vi "Repeat_Meas_if_Unsteady.vi"() -> (5 "Plug in titles":string[](array[string]), 7 "Plug in values":string[](array[string]))   [LabVIEW 2014]
uses:
  Controls/Post_Process.ctl
  Globals/Meas_global.vi
  <vilib>/Analysis/NI_AALPro.lvlib
panel:
  out "Waveform Graph":cluster{dbl, dbl, "Downsampled Array":dbl[][]}(graph)
  out "Repeat Measurement":bool
  in  "Minumum value to divide by":dbl=100.0 format="%#_13g"
  in  "Acceptable % Drift":dbl=0.8 format="%#_13g"
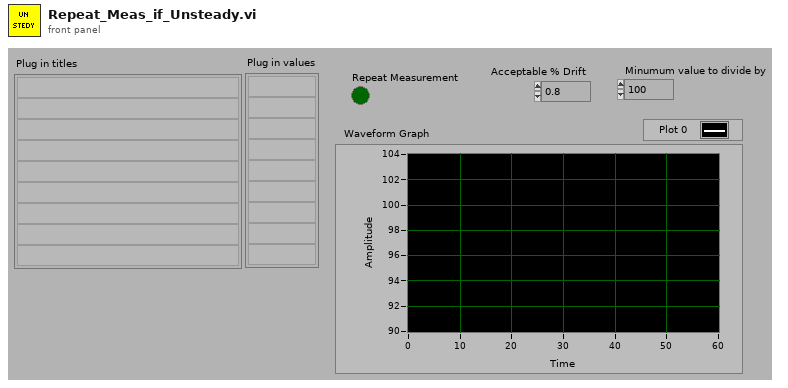
[diagram p1: front panel]
types:
  T1 = typedef "Analysis_info_cluster.ctl" = cluster{"Colour":u32, "Inst type":T2, "Inst name":string, "Symbol":string, "Code name":string, "Extra Info":string, "Inst Array":T3, "Extra Titles":string[], "Extra Values":string[], "U":dbl, "u^2":dbl, "u^3":dbl, "u^4":dbl, "Skew_u":dbl, "Kurt_u":dbl, "Sd Error in Mean":dbl, "% u'/U":dbl, "X":dbl, "Y":dbl, "Z":dbl, "Timescale integral to 25%":dbl, "Sd Error in Variance":dbl, "Calib File":path, "Calib Constants":dbl[], "Output Position":bool, "Full Stats":bool, "Av Sampling Rate":dbl, "Av No of Samples":dbl, "Total Meas Time (s)":dbl, "ADAM Ch Name":string}
  T2 = typedef "Inst_type.ctl" = enum16{"Propeller anemometer", "Raw voltage", "Pressure Transducer", "Pitot-static tube", "Preston tube", "Hot wire", "Cross wire 1", "Cross wire 2", "Generic Linear", "Generic Polynomial", "Generic BackPoly", "Fast FID", "Thermocouple", "Cold wire", "Pulsed Wire", "LDA Vel", "LDA Tran time", "LDA Arr time"}
  T3 = typedef "Instrument_Array.ctl" = enum16{"PWA", "LDA", "Analogue"}
  T4 = typedef "Time_Trace_Cluster.ctl" = cluster{"Weighting":dbl[], "Time (s)":dbl[], "Voltage":dbl[], "Eng Values":dbl[]}
  T5 = typedef "Post_Process.ctl" = enum16{"Take New Data", "Post Process Raw Data File"}
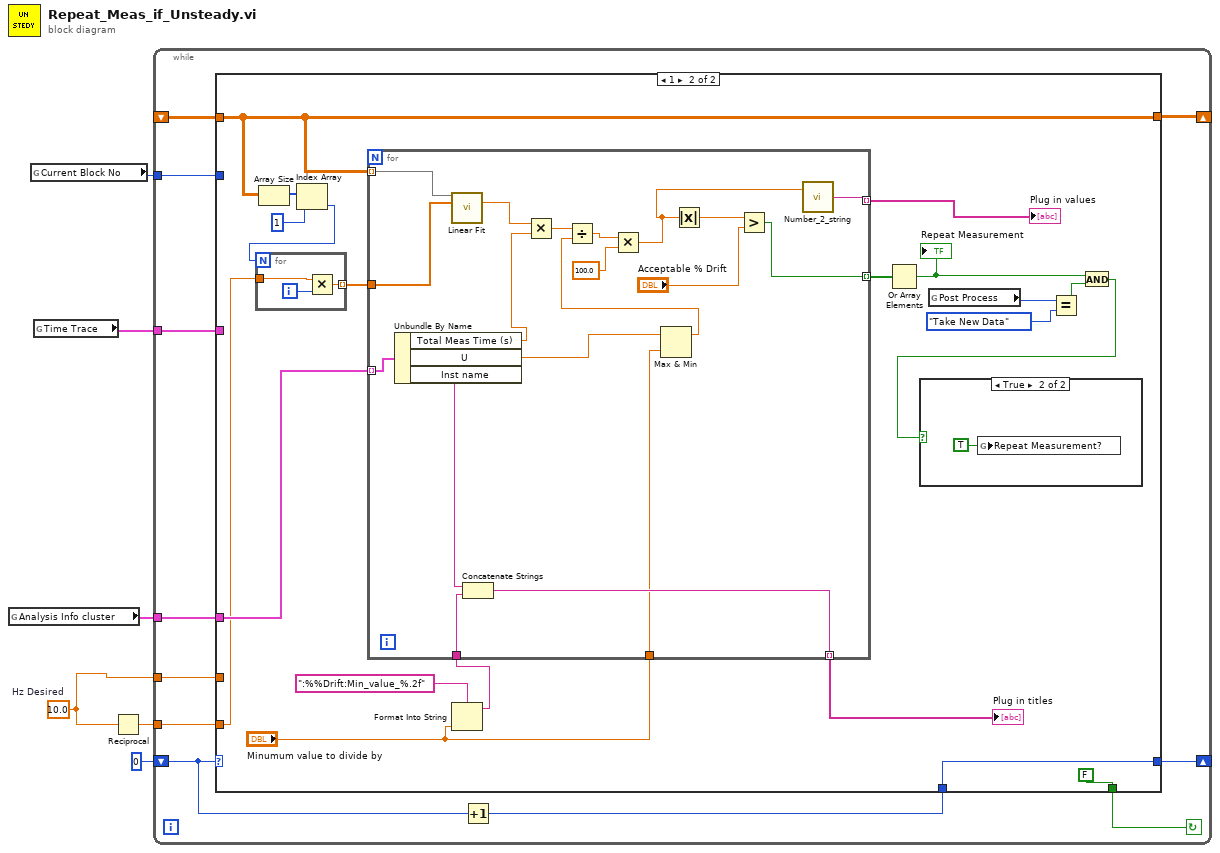
[diagram p0: block diagram]
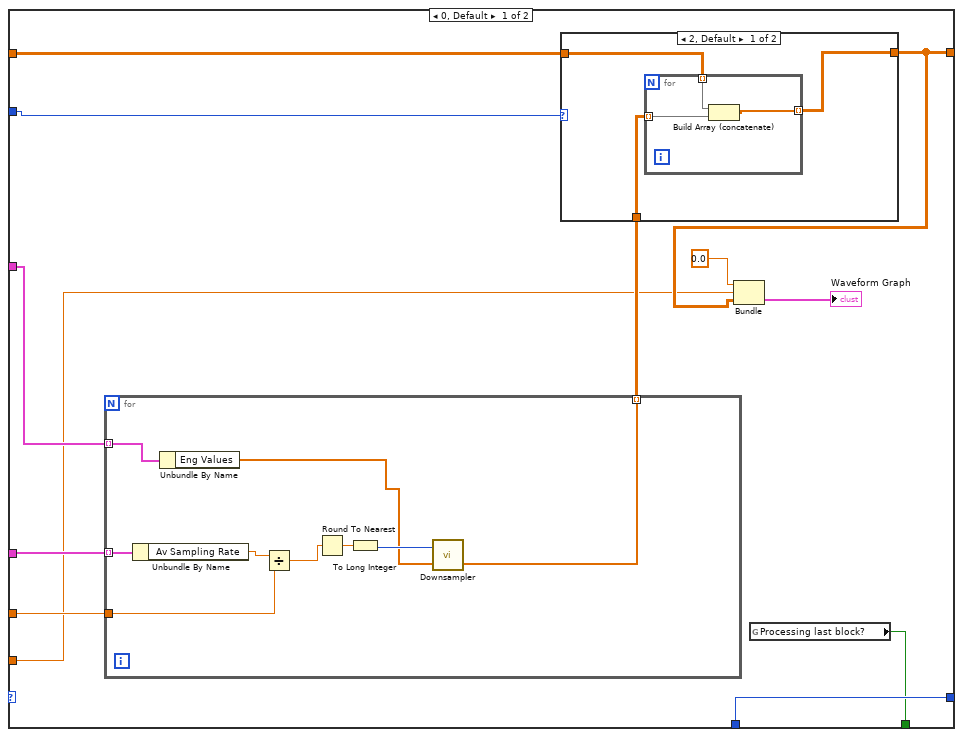
[diagram p2: hidden frame]
diagram:
  w2 = 10.0  # Hz Desired
  n1 = global read "Meas_global.vi" "Analysis Info cluster"() -> (w4:T1[])
  n2 = global read "Meas_global.vi" "Current Block No"() -> (w6:i32)
  n3 = global read "Meas_global.vi" "Time Trace"() -> (w3:T4[])
  n4 = Reciprocal(x=w2) -> (1/x=w1:dbl)
  n5 = while {
    shift-left: _ -> [w11]
    shift-right: [w12] -> _
    shift-left: 0 -> [w16]
    shift-right: [w14] -> _
    tunnel: w6 -> [w17]
    tunnel: w4 -> [w10]
    tunnel: w3 -> [w9]
    tunnel: w2 -> [w8]
    tunnel: w1 -> [w7]
    stop <- w13 continue-if-true
    n6 = Increment(x=w16) -> (x+1=w15:i32)
    n7 = case shown="1" w16 {
      tunnel: w17 -> [w28 _]
      tunnel: w15 -> [w29 w64]
      tunnel: [w29 w64] -> w14
      tunnel: [w24 FALSE] -> w13
      tunnel: [w21 w62] -> w12
      tunnel: w11 -> [w23 w62]
      tunnel: w10 -> [w27 w63]
      tunnel: w9 -> [w26 _]
      tunnel: w8 -> [w19 _]
      tunnel: w7 -> [w18 w51]
      frame 0, Default {
        n8 = for {
          tunnel: w27 -> [w38] mode=indexing
          tunnel: w26 -> [w37] mode=indexing
          tunnel: [w31] -> w25 mode=indexing
          tunnel: w19 -> [w30]
          n9 = Unbundle By Name(w38) -> ("Av Sampling Rate"=w36:dbl)
          n10 = Unbundle By Name(w37) -> ("Eng Values"=w32:dbl[])
          n11 = Divide(x=w36, y=w30) -> (x/y=w35:dbl)
          n12 = Round To Nearest(number=w35) -> (nearest integer value=w34:dbl)
          n13 = To Long Integer(number=w34) -> (32bit integer=w33:i32)
          n14 = call "Downsampler.vi"("Input Array"=w32, "Averaging samples"=w33) -> ("Downsampled Array"=w31:dbl[])  [unwired: 1 out]
        }
        n15 = case shown="2, Default" w28 {
          tunnel: [w39 w45] -> w21
          tunnel: w23 -> [w41 _]
          tunnel: w25 -> [w40 w45]
          frame 2, Default {
            n16 = for {
              tunnel: w41 -> [w44] mode=indexing
              tunnel: w40 -> [w43] mode=indexing
              tunnel: [w42] -> w39 mode=indexing
              n17 = Build Array (concatenate)(w44, w43) -> (w42:dbl[])
            }
          }
          frame 1 {
          }
        }
        n18 = Bundle(0.0, w18, "Downsampled Array"=w21) -> (→"Waveform Graph":cluster{dbl, dbl, "Downsampled Array":dbl[][]})  [unwired: 1 in]
        n19 = global read "Meas_global.vi" "Processing last block?"() -> (w24:bool)
      }
      frame 1 {
        n20 = Array Size(array=w62) -> (size(s)=w61:i32[])
        n21 = Index Array(array=w61, index=1) -> (element=w59:i32)
        n22 = for {
          N: w59 -> [_]
          tunnel: [w68] -> w58 mode=indexing
          tunnel: w51 -> [w67]
          i -> [w69]
          n23 = Multiply(x=w67, y=w69) -> (x*y=w68:dbl)
        }
        n24 = Format Into String(format string=":%%Drift:Min_value_%.2f", "Minumum value to divide by") -> (resulting string=w52:string)  [unwired: 2 in, 1 out]
        n25 = for {
          tunnel: w63 -> [w88] mode=indexing
          tunnel: [w86] -> w57 mode=indexing
          tunnel: w62 -> [w80] mode=indexing
          tunnel: [w85] -> w56 mode=indexing
          tunnel: w58 -> [w84]
          tunnel: w52 -> [w81]
          tunnel: [w71] -> w55 mode=indexing
          tunnel: "Minumum value to divide by" -> [w70]
          n26 = Unbundle By Name(w88) -> ("Total Meas Time (s)"=w78:dbl, "U"=w83:dbl, "Inst name"=w87:string)
          n27 = call <vilib>:"Linear Fit.vi"("Y"=w80, "X"=w84) -> ("slope"=w79:dbl)  [unwired: 9 in, 4 out]
          n28 = Concatenate Strings(w87, w81) -> (w86:string)
          n29 = Multiply(x=w79, y=w78) -> (x*y=w77:dbl)
          n30 = Max & Min(x=w83, y=w70) -> (max(x,y)=w76:dbl)  [unwired: 1 out]
          n31 = Divide(x=w77, y=w76) -> (x/y=w75:dbl)
          n32 = Multiply(x=w75, y=100.0) -> (x*y=w73:dbl)
          n33 = Absolute Value(x=w73) -> (abs(x)=w82:dbl)
          n34 = Greater?(x=w82, y="Acceptable % Drift") -> (0:w71:bool)
          n35 = call "Number_2_string.vi"("number"=w73) -> ("String"=w85:string)  [unwired: 1 in]
        }
        "Plug in titles" <- w57
        "Plug in values" <- w56
        n36 = Or Array Elements(Boolean array=w55) -> (logical OR=w47:bool)
        "Repeat Measurement" <- w47
        n37 = global read "Meas_global.vi" "Post Process"() -> (w49:T5)
        n38 = Equal?(x=w49, y=Post_Process."Take New Data" ("Post Process")) -> (x = y?=w48:bool)
        n39 = And(x=w47, y=w48) -> (x .and. y?=w46:bool)
        n40 = case shown="True" w46 {
          frame False {
          }
          frame True {
            n41 = global write "Meas_global.vi" "Repeat Measurement?"(TRUE ("Repeat Measurement?")) -> ()
          }
        }
      }
    }
  }
